vi "Launch Servo Motor.vi"() -> ()   [LabVIEW 2020]
uses:
  Device Manager/Device Manager/Device Manager.lvclass
  <vilib>/ActorFramework/Stop Msg/Stop Msg.lvclass
  <vilib>/ActorFramework/Actor/Actor.lvclass
panel:
  in  "Panel Port":refnum<visa-resource-name>
  in  "Motor Port":refnum<visa-resource-name>
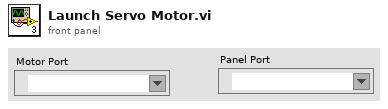
[diagram p1: front panel]
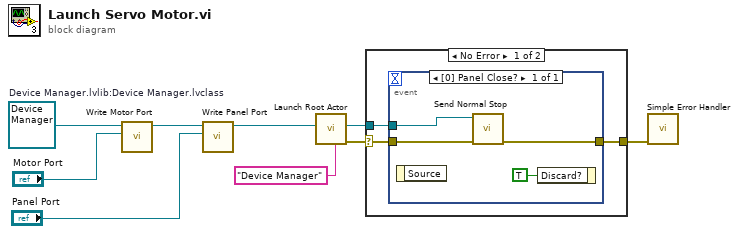
[diagram p0: block diagram]
diagram:
  w5 = refnum<class "Device Manager.lvclass"> refnum  # Device Manager.lvlib:Device Manager.lvclass
  n1 = call-dynamic "Write Motor Port.vi"("Motor Port"="Motor Port", "Device Manager in"=w5) -> ("Device Manager out"=w2:refnum<class "Device Manager.lvclass">)  [unwired: 9 in]
  n2 = call-dynamic "Write Panel Port.vi"("Panel Port"="Panel Port", "Device Manager in"=w2) -> ("Device Manager out"=w4:refnum<class "Device Manager.lvclass">)  [unwired: 9 in]
  n3 = call <vilib>:"Launch Root Actor.vi"("Debug Alias"="Device Manager", "Actor"=w4) -> ("error out"=w9:errorcluster, "Actor's Enqueuer"=w8:refnum<class "Message Enqueuer.lvclass">)  [unwired: 8 in]
  n4 = case shown="No Error" w9 {
    selector: w9 -> [w12 w17]
    tunnel: w8 -> [w11 _]
    tunnel: [w10 w17] -> w7
    frame No Error {
      n5 = event shown="[0] Panel Close?" {
        selector: _ -> [_]
        dyn-events: _ -> [_]
        timeout: _ -> [_]
        tunnel: w12 -> [w15]
        tunnel: w11 -> [w14]
        tunnel: [w13] -> w10
        event Panel Close? {
          n6 = event-data() -> ()  [unwired: 1 in, 1 out]
          n7 = call <vilib>:"Send Normal Stop.vi"("error in (no error)"=w15, "Message Enqueuer"=w14) -> ("error out"=w13:errorcluster)  [unwired: 9 in]
          n8 = event-data("Discard?"=TRUE) -> ()  [unwired: 1 in, 1 out]
        }
      }
    }
    frame Error {
    }
  }
  n9 = call <vilib>:"Simple Error Handler.vi"("error in (no error)"=w7) -> ()  [unwired: 4 in, 5 out]
